vi "Basic Constructor.vi"(6 "Nested panels for additional? (T)":bool=TRUE, 7 "Nested panels for root? (F)":bool, 8 "error in (no error)":errorcluster, 9 "Additional Panels (window)":refnum<class "Panel.lvclass">, 10 "Root Panel":refnum<class "Panel.lvclass">, 11 "Model Panel Logic in":refnum<class "Model Panel Logic Nested Window.lvclass">) -> (0 "error out":errorcluster, 3 "Model Panel Logic out":refnum<class "Model Panel Logic Nested Window.lvclass">)   [LabVIEW 2020, in "Form Model.lvlib" / "Model Panel Logic Nested Window.lvclass"]
uses:
  Model Panel Logic Nested Window.lvclass
  <vilib>/MGI/Panel Manager/Panel/Panel/Panel.lvclass
  Model Panel Logic Nested Window.lvclass/Model Panel Logic Nested Window.ctl
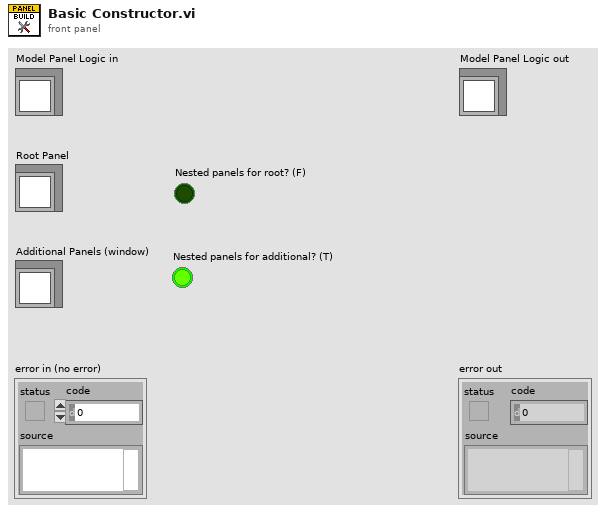
[diagram p1: front panel]
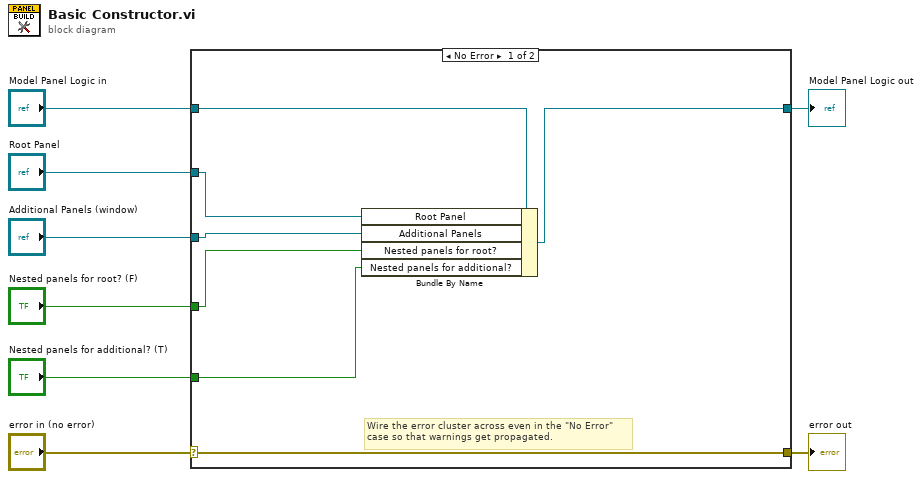
[diagram p0: block diagram]
diagram:
  n1 = case shown="No Error" "error in (no error)" {
    selector: "error in (no error)" -> [w15 w17]
    tunnel: [w15 w17] -> w7
    tunnel: [w13 w16] -> w5
    tunnel: "Model Panel Logic in" -> [w14 w16]
    tunnel: "Root Panel" -> [w12 _]
    tunnel: "Additional Panels (window)" -> [w11 _]
    tunnel: "Nested panels for root? (F)" -> [w10 _]
    tunnel: "Nested panels for additional? (T)" -> [w9 _]
    frame No Error {
      # "Wire the error cluster across even in the \"No Error\"\ncase so that warnings get propagated."
      n2 = Bundle By Name(cluster=w14, "Root Panel"=w12, "Additional Panels"=w11, "Nested panels for root?"=w10, "Nested panels for additional?"=w9) -> (w13:refnum<class "Model Panel Logic Nested Window.lvclass">)
    }
    frame Error {
    }
  }
  "error out" <- w7
  "Model Panel Logic out" <- w5
